vi "start_warning.vi"(8 "error in":errorcluster) -> (0 "error out":errorcluster, 3 "Cancelado?":bool)   [LabVIEW 2016]
panel:
  in  "Cancel":bool
  in  "OK":bool
  out "Info":string
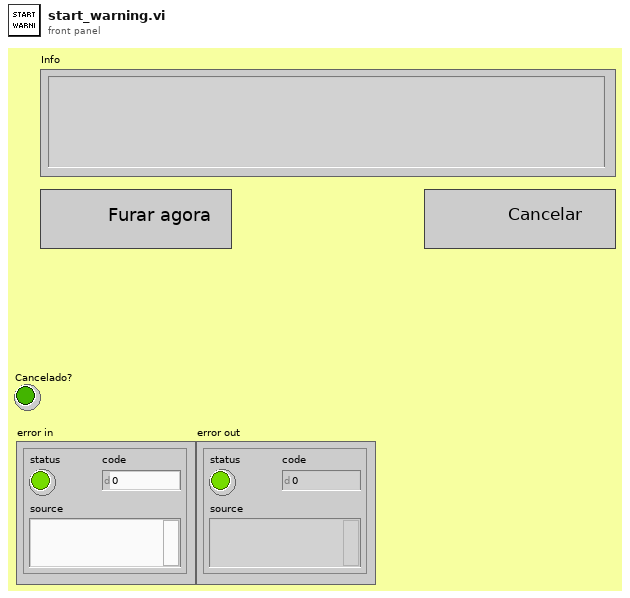
[diagram p1: front panel]
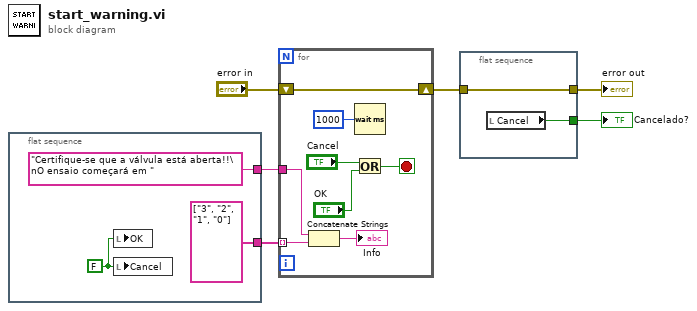
[diagram p0: block diagram]
diagram:
  n1 = flat-sequence {
    tunnel: ["Certifique-se que a válvula está aberta!!\nO ensaio começará em " ("Info")] -> w6
    tunnel: [string[] ["3", "2", "1", "0"]] -> w5
    frame #0 {
      w7 = FALSE ("OK")
      n2 = local write "OK"(w7) -> ()
      n3 = local write "Cancel"(w7) -> ()
    }
  }
  n4 = for {
    tunnel: w6 -> [w16]
    tunnel: w5 -> [w15] mode=indexing
    shift-right: [w10] -> w3
    shift-left: "error in" -> [w10]
    stop <- w13 stop-if-true
    n5 = Concatenate Strings(w16, w15) -> (→"Info":string)
    n6 = Wait (ms)(milliseconds to wait=u32 1000) -> ()  [unwired: 1 out]
    n7 = Or(x="Cancel", y="OK") -> (x .or. y?=w13:bool)
  }
  n8 = flat-sequence {
    tunnel: w3 -> [w19]
    tunnel: [w19] -> w2
    tunnel: [w18] -> w1
    frame #0 {
      n9 = local read "Cancel"() -> (w18:bool)
    }
  }
  "Cancelado?" <- w1
  "error out" <- w2
